vi "FFTtoR,Theta (2D).VI"(0 "X":dbl[][](array[numeric]) format="%.2f") -> (1 "+Freq. Mag of FFT":dbl[][](array[numeric]) min=0.0 max=127.0 format="%.2f", 2 "+Freq Theta of FFT":dbl[][](array[numeric]) min=0.0 max=127.0 format="%.2f")   [LabVIEW 2020]
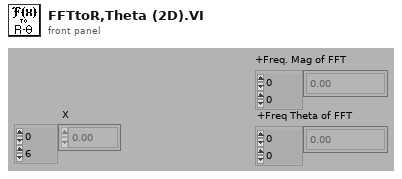
[diagram p1: front panel]
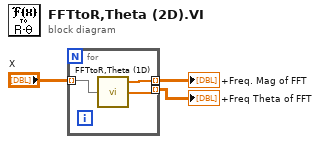
[diagram p0: block diagram]
diagram:
  n1 = for {
    tunnel: "X" -> [w6] mode=indexing
    tunnel: [w5] -> w2 mode=indexing
    tunnel: [w4] -> w3 mode=indexing
    n2 = call "FFTtoR,Theta (1D).VI"("X"=w6) -> ("+Freq. Mag of FFT"=w5:dbl[], "+Freq Theta of FFT"=w4:dbl[])  [unwired: 1 in]
  }
  "+Freq. Mag of FFT" <- w2
  "+Freq Theta of FFT" <- w3
